vi "Send.vi"(10 "Queue Actor":refnum<class "Queue Actor.lvclass">) -> (3 "Queue Last Ack Msg out":refnum<class "Queue Last Ack Msg.lvclass">)   [LabVIEW 2021, in "Queue Last Ack.lvlib" / "Queue Last Ack Msg.lvclass"]
uses:
  Queue Last Ack Msg.lvclass
  Queue Actor/Queue Actor.lvclass
  Queue Last Ack Msg.lvclass/Queue Last Ack Msg.ctl
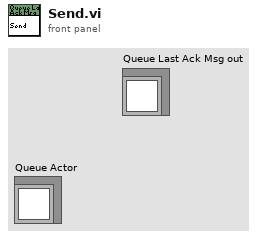
[diagram p1: front panel]
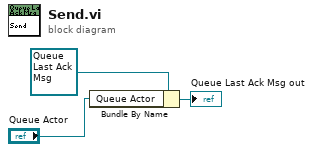
[diagram p0: block diagram]
diagram:
  n1 = Bundle By Name(cluster=refnum<class "Queue Last Ack Msg.lvclass"> refnum ("Last Ack Msg in"), "Queue Actor"="Queue Actor") -> (→"Queue Last Ack Msg out":refnum<class "Queue Last Ack Msg.lvclass">)
